vi "DeviceLookup.vi"(4 "error in (no error)":errorcluster, 7 "report in":refnum<class "NI_report.lvclass">) -> (0 "error out":errorcluster, 1 "report out":refnum<class "NI_report.lvclass">, 2 "[[DeviceTypesVals]]":i32[][](array[numeric]), 3 "[[Device Types]]":string[][](array[string]))   [LabVIEW 2013]
uses:
  <vilib>/Utility/NIReport.llb/NI_report.lvclass
  <vilib>/addons/_office/excel.llb/Excel Get Data ([str]).vi
  <vilib>/addons/_office/excel.llb/Excel Get Data ([i32]).vi
  <vilib>/addons/_office/NI_ReportGenerationToolkit.lvlib
  <vilib>/Utility/NIReport.llb/Excel/NI_Excel.lvclass
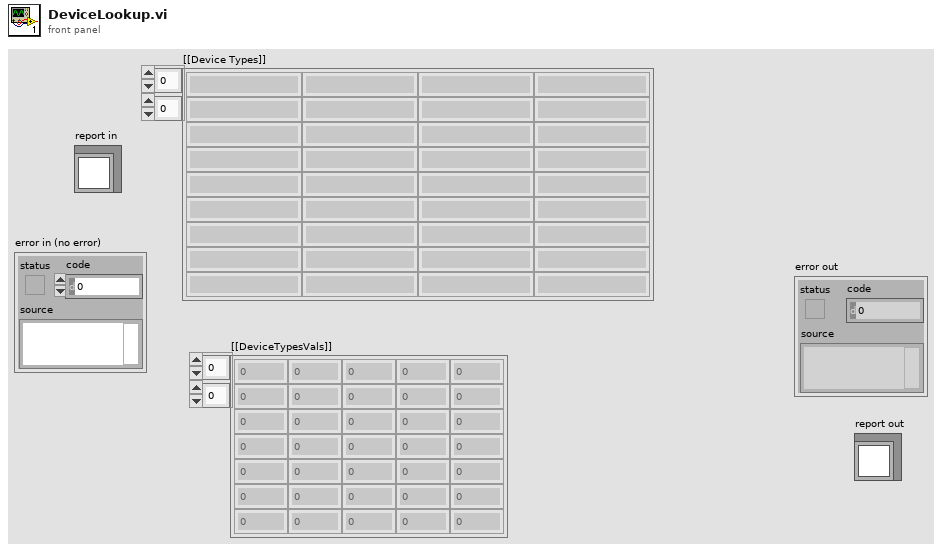
[diagram p1: front panel]
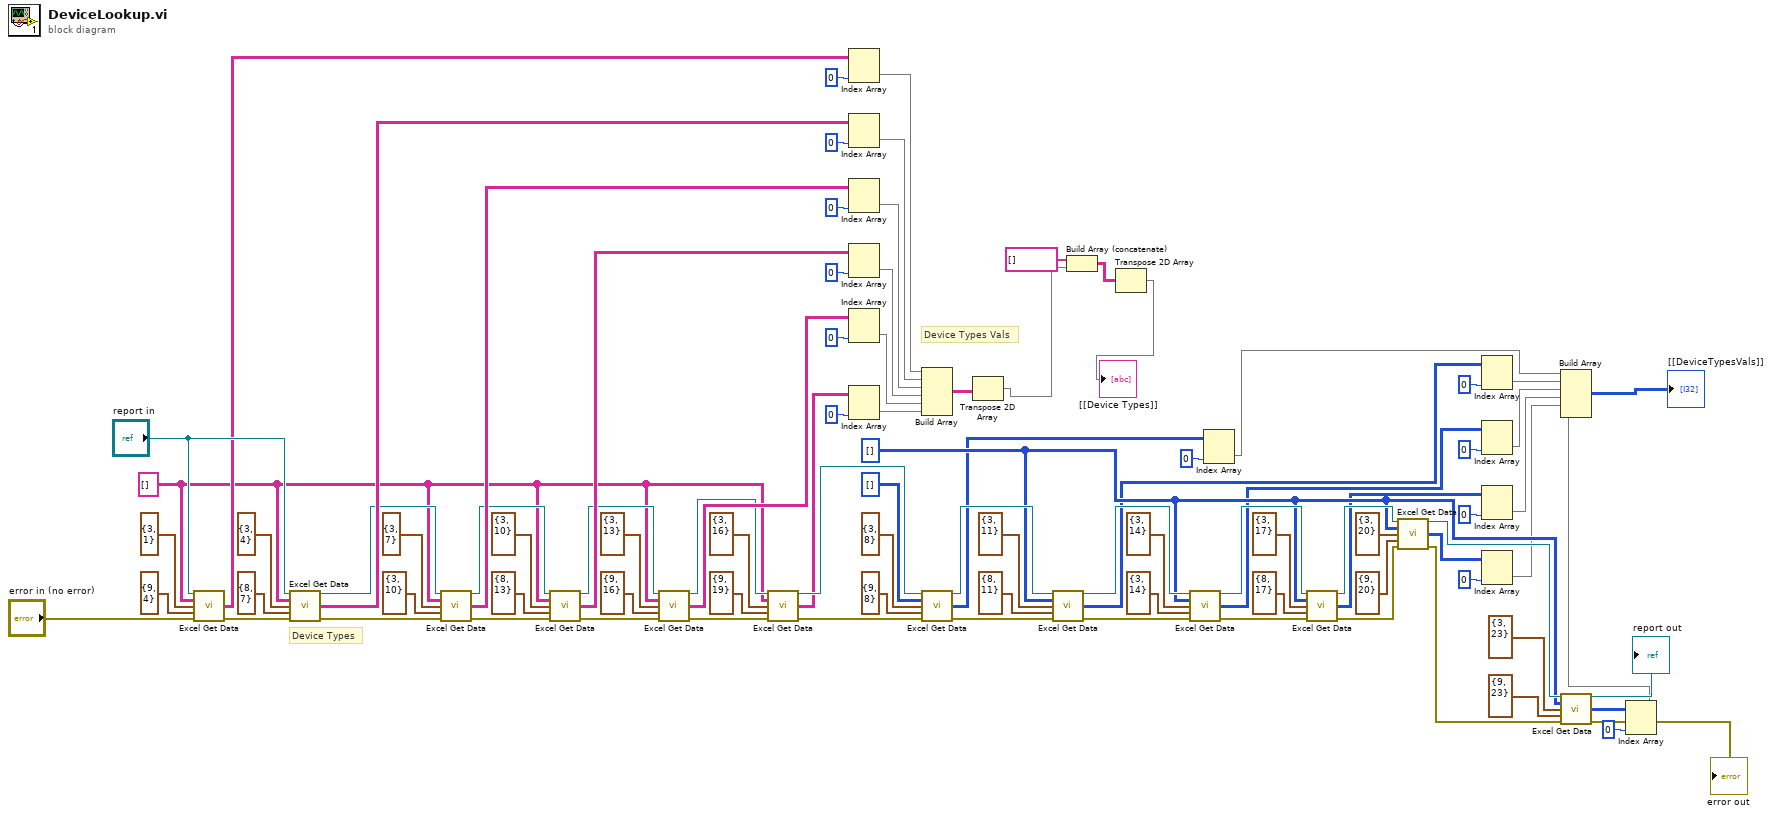
[diagram p0: block diagram]
diagram:
  w31 = i32[][] [] ("data type")
  w58 = string[][] [] ("data type")
  # "Device Types Vals"
  # "Device Types"
  n1 = call-poly <vilib>:"Excel Get Data.vi"("report in"="report in", "data type"=w58, "start (-1, -1)"=cluster{"row":i32, "column":i32} {"row"=3, "column"=1}, "end (-1, -1)"=cluster{"row":i32, "column":i32} {"row"=9, "column"=4}, "error in (no error)"="error in (no error)") -> ("data"=w87:string[][], "error out"=w88:errorcluster)  [unwired: 8 in, 1 out]
  n2 = call-poly <vilib>:"Excel Get Data.vi"("report in"="report in", "data type"=w58, "start (-1, -1)"=cluster{"row":i32, "column":i32} {"row"=3, "column"=4}, "end (-1, -1)"=cluster{"row":i32, "column":i32} {"row"=8, "column"=7}, "error in (no error)"=w88) -> ("report out"=w81:refnum<class "NI_report.lvclass">, "data"=w84:string[][], "error out"=w80:errorcluster)  [unwired: 8 in]
  n3 = call-poly <vilib>:"Excel Get Data.vi"("report in"=w81, "data type"=w58, "start (-1, -1)"=cluster{"row":i32, "column":i32} {"row"=3, "column"=7}, "end (-1, -1)"=cluster{"row":i32, "column":i32} {"row"=3, "column"=10}, "error in (no error)"=w80) -> ("report out"=w74:refnum<class "NI_report.lvclass">, "data"=w76:string[][], "error out"=w73:errorcluster)  [unwired: 8 in]
  n4 = call-poly <vilib>:"Excel Get Data.vi"("report in"=w74, "data type"=w58, "start (-1, -1)"=cluster{"row":i32, "column":i32} {"row"=3, "column"=10}, "end (-1, -1)"=cluster{"row":i32, "column":i32} {"row"=8, "column"=13}, "error in (no error)"=w73) -> ("report out"=w67:refnum<class "NI_report.lvclass">, "data"=w69:string[][], "error out"=w66:errorcluster)  [unwired: 8 in]
  n5 = call-poly <vilib>:"Excel Get Data.vi"("report in"=w67, "data type"=w58, "start (-1, -1)"=cluster{"row":i32, "column":i32} {"row"=3, "column"=13}, "end (-1, -1)"=cluster{"row":i32, "column":i32} {"row"=9, "column"=16}, "error in (no error)"=w66) -> ("report out"=w59:refnum<class "NI_report.lvclass">, "data"=w62:string[][], "error out"=w60:errorcluster)  [unwired: 8 in]
  n6 = call-poly <vilib>:"Excel Get Data.vi"("report in"=w59, "data type"=w58, "start (-1, -1)"=cluster{"row":i32, "column":i32} {"row"=3, "column"=16}, "end (-1, -1)"=cluster{"row":i32, "column":i32} {"row"=9, "column"=19}, "error in (no error)"=w60) -> ("report out"=w55:refnum<class "NI_report.lvclass">, "data"=w11:string[][], "error out"=w54:errorcluster)  [unwired: 8 in]
  n7 = Index Array(array=w87, index (col)=0 ("disabled index (col)")) -> (element=w83:string[])  [unwired: 1 in]
  n8 = Index Array(array=w84, index (col)=0 ("disabled index (col)")) -> (element=w82:string[])  [unwired: 1 in]
  n9 = Index Array(array=w76, index (col)=0 ("disabled index (col)")) -> (element=w75:string[])  [unwired: 1 in]
  n10 = Index Array(array=w69, index (col)=0 ("disabled index (col)")) -> (element=w68:string[])  [unwired: 1 in]
  n11 = Index Array(array=w62, index (col)=0 ("disabled index (col)")) -> (element=w61:string[])  [unwired: 1 in]
  n12 = Index Array(array=w11, index (col)=0 ("disabled index (col)")) -> (element=w10:string[])  [unwired: 1 in]
  n13 = Build Array(w83, w82, w75, w68, w61, w10) -> (w6:string[][])
  n14 = call-poly <vilib>:"Excel Get Data.vi"("report in"=w55, "data type"=i32[][] [], "start (-1, -1)"=cluster{"row":i32, "column":i32} {"row"=3, "column"=8}, "end (-1, -1)"=cluster{"row":i32, "column":i32} {"row"=9, "column"=8}, "error in (no error)"=w54) -> ("report out"=w48:refnum<class "NI_report.lvclass">, "data"=w28:i32[][], "error out"=w47:errorcluster)  [unwired: 8 in]
  n15 = Transpose 2D Array(2D array=w6) -> (transposed array=w5:string[][])
  n16 = call-poly <vilib>:"Excel Get Data.vi"("report in"=w48, "data type"=w31, "start (-1, -1)"=cluster{"row":i32, "column":i32} {"row"=3, "column"=11}, "end (-1, -1)"=cluster{"row":i32, "column":i32} {"row"=8, "column"=11}, "error in (no error)"=w47) -> ("report out"=w44:refnum<class "NI_report.lvclass">, "data"=w26:i32[][], "error out"=w43:errorcluster)  [unwired: 8 in]
  n17 = Build Array (concatenate)(string[] [] ("element"), w5) -> (w2:string[][])
  n18 = Transpose 2D Array(2D array=w2) -> (transposed array=→"[[Device Types]]":string[][])
  n19 = call-poly <vilib>:"Excel Get Data.vi"("report in"=w44, "data type"=w31, "start (-1, -1)"=cluster{"row":i32, "column":i32} {"row"=3, "column"=14}, "end (-1, -1)"=cluster{"row":i32, "column":i32} {"row"=3, "column"=14}, "error in (no error)"=w43) -> ("report out"=w39:refnum<class "NI_report.lvclass">, "data"=w23:i32[][], "error out"=w40:errorcluster)  [unwired: 8 in]
  n20 = Index Array(array=w28, index (col)=0 ("disabled index (col)")) -> (element=w17:i32[])  [unwired: 1 in]
  n21 = call-poly <vilib>:"Excel Get Data.vi"("report in"=w39, "data type"=w31, "start (-1, -1)"=cluster{"row":i32, "column":i32} {"row"=3, "column"=17}, "end (-1, -1)"=cluster{"row":i32, "column":i32} {"row"=8, "column"=17}, "error in (no error)"=w40) -> ("report out"=w36:refnum<class "NI_report.lvclass">, "data"=w22:i32[][], "error out"=w35:errorcluster)  [unwired: 8 in]
  n22 = call-poly <vilib>:"Excel Get Data.vi"("report in"=w36, "data type"=w31, "start (-1, -1)"=cluster{"row":i32, "column":i32} {"row"=3, "column"=20}, "end (-1, -1)"=cluster{"row":i32, "column":i32} {"row"=9, "column"=20}, "error in (no error)"=w35) -> ("report out"=w32:refnum<class "NI_report.lvclass">, "data"=w20:i32[][], "error out"=w30:errorcluster)  [unwired: 8 in]
  n23 = Index Array(array=w26, index (col)=0 ("disabled index (col)")) -> (element=w16:i32[])  [unwired: 1 in]
  n24 = Index Array(array=w23, index (col)=0 ("disabled index (col)")) -> (element=w15:i32[])  [unwired: 1 in]
  n25 = Index Array(array=w22, index (col)=0 ("disabled index (col)")) -> (element=w14:i32[])  [unwired: 1 in]
  n26 = Index Array(array=w20, index (col)=0 ("disabled index (col)")) -> (element=w13:i32[])  [unwired: 1 in]
  n27 = call-poly <vilib>:"Excel Get Data.vi"("report in"=w32, "data type"=w31, "start (-1, -1)"=cluster{"row":i32, "column":i32} {"row"=3, "column"=23}, "end (-1, -1)"=cluster{"row":i32, "column":i32} {"row"=9, "column"=23}, "error in (no error)"=w30) -> ("report out"=→"report out":refnum<class "NI_report.lvclass">, "data"=w18:i32[][], "error out"=→"error out":errorcluster)  [unwired: 8 in]
  n28 = Index Array(array=w18, index (col)=0 ("disabled index (col)")) -> (element=w1:i32[])  [unwired: 1 in]
  n29 = Build Array(w17, w16, w15, w14, w13, w1) -> (→"[[DeviceTypesVals]]":i32[][])
